vi "Set OD Index.vi"(8 "error in (no error)":errorcluster, 10 "OD Index":u16 format="%.0x", 11 "PDO Communication Parameter in":refnum<class "PDO Communication Parameter.lvclass">) -> (0 "error out":errorcluster, 3 "PDO Communication Parameter out":refnum<class "PDO Communication Parameter.lvclass">)   [LabVIEW 2024, in "PDO Grid.lvlib" / "PDO Communication Parameter.lvclass"]
uses:
  PDO Communication Parameter.lvclass
  PDO Communication Parameter.lvclass/PDO Communication Parameter.ctl
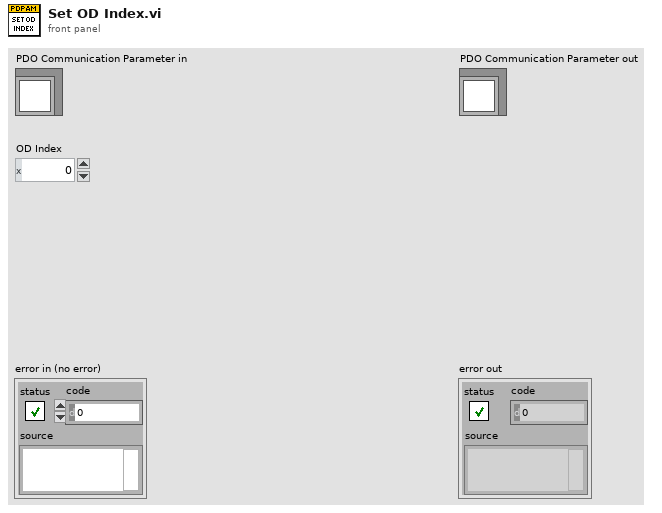
[diagram p1: front panel]
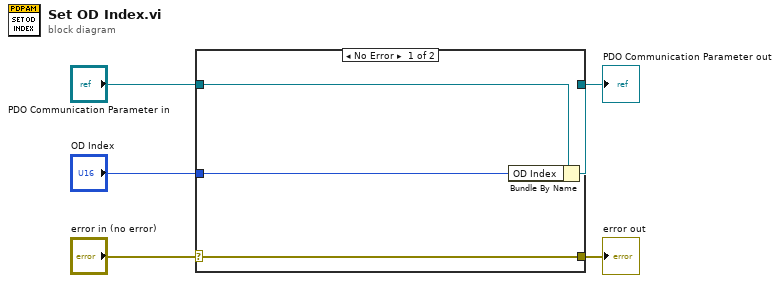
[diagram p0: block diagram]
diagram:
  n1 = case shown="No Error" "error in (no error)" {
    selector: "error in (no error)" -> [w9 w10]
    tunnel: [w9 w10] -> w4
    tunnel: [w7 w11] -> w2
    tunnel: "PDO Communication Parameter in" -> [w8 w11]
    tunnel: "OD Index" -> [w6 _]
    frame No Error {
      n2 = Bundle By Name(cluster=w8, "OD Index"=w6) -> (w7:refnum<class "PDO Communication Parameter.lvclass">)
    }
    frame Error {
    }
  }
  "error out" <- w4
  "PDO Communication Parameter out" <- w2
